vi "MQTT_Subscribe_Read.vi"(8 "error in (no error)":errorcluster, 10 "Bytes Read":u8[](array[numeric]) format="%x") -> (0 "error out":errorcluster, 2 "Subscription Info Array":cluster{"Topic":string, "QoS":T1}[](array[cluster])=[{"Topic"="a/b", "QoS"=enum."At least once"}])   [LabVIEW 2012, in "MQTT_Functions.lvlib"]
uses:
  MQTT_Functions.lvlib
  Controls/QoS.ctl
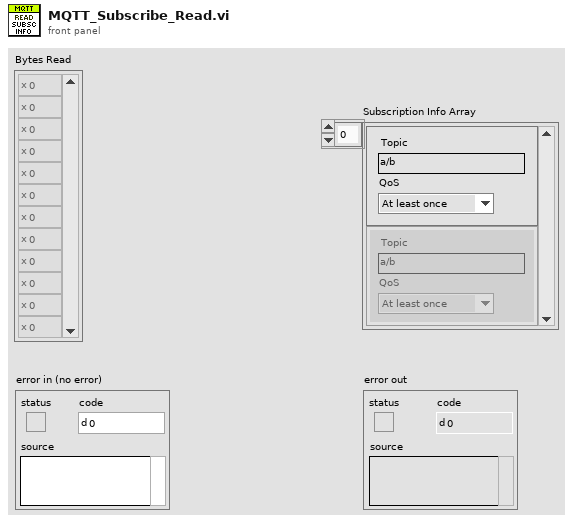
[diagram p1: front panel]
types:
  T1 = typedef "MQTT_Functions.lvlib/QoS.ctl" = enum8{"At most once", "At least once", "Exactly once", "Reserved"}
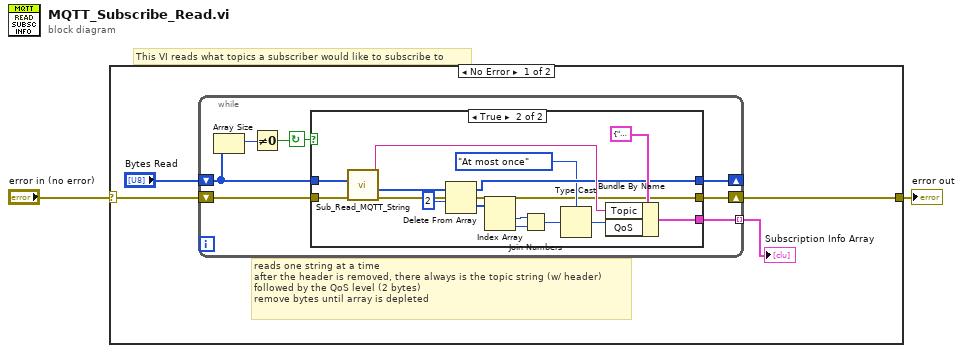
[diagram p0: block diagram]
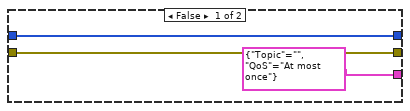
[diagram p2: hidden frame]
diagram:
  # "This VI reads what topics a subscriber would like to subscribe to"
  n1 = case shown="No Error" "error in (no error)" {
    selector: "error in (no error)" -> [w5 w32]
    tunnel: [w3 w32] -> w1
    frame No Error {
      # "reads one string at a time\nafter the header is removed, there always is the topic string (w/ header) \nfollowed by the QoS level (2 bytes)\nremove bytes until array is depleted"
      n2 = while {
        shift-right: [w12] -> _
        shift-left: "Bytes Read" -> [w9]
        tunnel: [w11] -> w4 mode=indexing
        shift-right: [w10] -> w3
        shift-left: w5 -> [w13]
        stop <- w7 continue-if-true
        n3 = Array Size(array=w9) -> (size(s)=w8:i32)
        n4 = Not Equal To 0?(x=w8) -> (x != 0?=w7:bool)
        n5 = case shown="True" w7 {
          tunnel: w13 -> [w15 w31]
          tunnel: [w16 w27] -> w12
          tunnel: [cluster{"Topic":string, "QoS":T1} {"Topic"="", "QoS"=enum."At most once"} ("Subscription Info") w19] -> w11
          tunnel: [w15 w18] -> w10
          tunnel: w9 -> [w16 w17]
          frame False {
          }
          frame True {
            n6 = call "Sub_Read_MQTT_String.vi"("error in (no error)"=w31, "UTF8 Byte Array"=w17) -> ("error out"=w18:errorcluster, "remaining bytes"=w28:u8[], "String"=w29:string)  [unwired: 7 in]
            n7 = Delete From Array(array=w28, length=2) -> (deleted portion=w25:u8[], array with subset deleted=w27:u8[])  [unwired: 1 in]
            n8 = Index Array(array=w25) -> (element #1=w24:u8, element #2=w23:u8)  [unwired: 2 in]
            n9 = Join Numbers(hi=w24, lo=w23) -> ((hi.lo)=w22:u16)
            n10 = Type Cast(type=QoS."At most once" ("QoS"), x=w22) -> (*(type *) &x=w20:T1)
            n11 = Bundle By Name(cluster=cluster{"Topic":string, "QoS":T1} {"Topic"="a/b", "QoS"=enum."At least once"} ("Subscription Info"), "Topic"=w29, "QoS"=w20) -> (w19:cluster{"Topic":string, "QoS":T1})
          }
        }
      }
      "Subscription Info Array" <- w4
    }
    frame Error {
    }
  }
  "error out" <- w1
